vi "GeoData.vi"() -> ()   [LabVIEW 2017] (continued)
Ethridge\tTN\tGiles County\tH1\n38478\t47055\tPulaski\tTN\tGiles County\tH1\n38468\t47055\tLeoma\tTN\tGiles County\tH1\n38460\t47055\tGoodspring\tTN\tGiles County\tH1\n38477\t47055\tProspect\tTN\tGiles County\tH1\n37047\t47055\tCornersville\tTN\tGiles County\tH1\n38472\t47055\tLynnville\tTN\tGiles County\tH1\n38459\t47055\tFrankewing\tTN\tGiles County\tH1\n38451\t47055\tCulleoka\tTN\tGiles County\tH1\n38464\t47055\tLawrenceburg\tTN\tGiles County\tH1\n38483\t47055\tSummertown\tTN\tGiles County\tH1\n38473\t47055\tMinor hill\tTN\tGiles County\tH1\n38453\t47055\tDellrose\tTN\tGiles County\tH1\n38455\t47055\tElkton\tTN\tGiles County\tH1\n37848\t47057\tPowder springs\tTN\tGrainger County\tH1\n37708\t47057\tBean station\tTN\tGrainger County\tH1\n37888\t47057\tWashburn\tTN\tGrainger County\tH1\n37861\t47057\tRutledge\tTN\tGrainger County\tH1\n37779\t47057\tLuttrell\tTN\tGrainger County\tH1\n37811\t47057\tMooresburg\tTN\tGrainger County\tH1\n37869\t47057\tSneedville\tTN\tGrainger County\tH1\n37709\t47057\tBlaine\tTN\tGrainger County\tH1\n37806\t47057\tMascot\tTN\tGrainger County\tH1\n37881\t47057\tThorn hill\tTN\tGrainger County\tH1\n37711\t47059\tBulls gap\tTN\tGreene County\tH1\n37810\t47059\tMohawk\tTN\tGreene County\tH1\n37641\t47059\tChuckey\tTN\tGreene County\tH1\n37745\t47059\tGreeneville\tTN\tGreene County\tH1\n37681\t47059\tLimestone\tTN\tGreene County\tH1\n37743\t47059\tGreeneville\tTN\tGreene County\tH1\n37616\t47059\tAfton\tTN\tGreene County\tH1\n37656\t47059\tFall branch\tTN\tGreene County\tH1\n37809\t47059\tMidway\tTN\tGreene County\tH1\n37857\t47059\tRogersville\tTN\tGreene County\tH1\n37818\t47059\tMosheim\tTN\tGreene County\tH1\n37365\t47061\tPalmer\tTN\tGrundy County\tH1\n37357\t47061\tMorrison\tTN\tGrundy County\tH1\n37397\t47061\tWhitwell\tTN\tGrundy County\tH1\n37366\t47061\tPelham\tTN\tGrundy County\tH1\n37339\t47061\tGruetli laager\tTN\tGrundy County\tH1\n37387\t47061\tTracy city\tTN\tGrundy County\tH1\n37313\t47061\tCoalmont\tTN\tGrundy County\tH1\n37374\t47061\tSequatchie\tTN\tGrundy County\tH1\n37356\t47061\tMonteagle\tTN\tGrundy County\tH1\n37110\t47061\tMcminnville\tTN\tGrundy County\tH1\n37301\t47061\tAltamont\tTN\tGrundy County\tH1\n37305\t47061\tBeersheba springs\tTN\tGrundy County\tH1\n37711\t47063\tBulls gap\tTN\tHamblen County\tH1\n37813\t47063\tMorristown\tTN\tHamblen County\tH1\n37877\t47063\tTalbott\tTN\tHamblen County\tH1\n37815\t47063\tMorristown\tTN\tHamblen County\tH1\n37891\t47063\tWhitesburg\tTN\tHamblen County\tH1\n37816\t47063\tMorristown\tTN\tHamblen County\tH1\n37814\t47063\tMorristown\tTN\tHamblen County\tH1\n37778\t47063\tLowland\tTN\tHamblen County\tH1\n37860\t47063\tRussellville\tTN\tHamblen County\tH1\n37890\t47063\tWhite pine\tTN\tHamblen County\tH1\n37341\t47065\tHarrison\tTN\tHamilton County\tH1\n37353\t47065\tMc donald\tTN\tHamilton County\tH1\n37379\t47065\tSoddy daisy\tTN\tHamilton County\tH1\n37311\t47065\tCleveland\tTN\tHamilton County\tH1\n37350\t47065\tLookout mountain\tTN\tHamilton County\tH1\n37338\t47065\tGraysville\tTN\tHamilton County\tH1\n37409\t47065\tChattanooga\tTN\tHamilton County\tH1\n37302\t47065\tApison\tTN\tHamilton County\tH1\n37416\t47065\tChattanooga\tTN\tHamilton County\tH1\n37421\t47065\tChattanooga\tTN\tHamilton County\tH1\n37450\t47065\tChattanooga\tTN\tHamilton County\tH1\n37308\t47065\tBirchwood\tTN\tHamilton County\tH1\n37403\t47065\tChattanooga\tTN\tHamilton County\tH1\n37406\t47065\tChattanooga\tTN\tHamilton County\tH1\n37410\t47065\tChattanooga\tTN\tHamilton County\tH1\n37415\t47065\tChattanooga\tTN\tHamilton County\tH1\n37404\t47065\tChattanooga\tTN\tHamilton County\tH1\n37304\t47065\tBakewell\tTN\tHamilton County\tH1\n37373\t47065\tSale creek\tTN\tHamilton County\tH1\n37402\t47065\tChattanooga\tTN\tHamilton County\tH1\n37405\t47065\tChattanooga\tTN\tHamilton County\tH1\n37401\t47065\tChattanooga\tTN\tHamilton County\tH1\n37315\t47065\tCollegedale\tTN\tHamilton County\tH1\n37407\t47065\tChattanooga\tTN\tHamilton County\tH1\n37384\t47065\tSoddy daisy\tTN\tHamilton County\tH1\n37336\t47065\tGeorgetown\tTN\tHamilton County\tH1\n37363\t47065\tOoltewah\tTN\tHamilton County\tH1\n37411\t47065\tChattanooga\tTN\tHamilton County\tH1\n37412\t47065\tChattanooga\tTN\tHamilton County\tH1\n37422\t47065\tChattanooga\tTN\tHamilton County\tH1\n37351\t47065\tLupton city\tTN\tHamilton County\tH1\n37343\t47065\tHixson\tTN\tHamilton County\tH1\n37377\t47065\tSignal mountain\tTN\tHamilton County\tH1\n37408\t47065\tChattanooga\tTN\tHamilton County\tH1\n37419\t47065\tChattanooga\tTN\tHamilton County\tH1\n37414\t47065\tChattanooga\tTN\tHamilton County\tH1\n37424\t47065\tChattanooga\tTN\tHamilton County\tH1\n37765\t47067\tKyles ford\tTN\tHancock County\tH1\n37731\t47067\tEidson\tTN\tHancock County\tH1\n37879\t47067\tTazewell\tTN\tHancock County\tH1\n37752\t47067\tHarrogate\tTN\tHancock County\tH1\n37869\t47067\tSneedville\tTN\tHancock County\tH1\n37881\t47067\tThorn hill\tTN\tHancock County\tH1\n38075\t47069\tWhiteville\tTN\tHardeman County\tH1\n38061\t47069\tPocahontas\tTN\tHardeman County\tH1\n38392\t47069\tMercer\tTN\tHardeman County\tH1\n38356\t47069\tMedon\tTN\tHardeman County\tH1\n38067\t47069\tSaulsbury\tTN\tHardeman County\tH1\n38039\t47069\tGrand junction\tTN\tHardeman County\tH1\n38042\t47069\tHickory valley\tTN\tHardeman County\tH1\n38340\t47069\tHenderson\tTN\tHardeman County\tH1\n38052\t47069\tMiddleton\tTN\tHardeman County\tH1\n38381\t47069\tToone\tTN\tHardeman County\tH1\n38008\t47069\tBolivar\tTN\tHardeman County\tH1\n38044\t47069\tHornsby\tTN\tHardeman County\tH1\n38371\t47071\tSardis\tTN\tHardin County\tH1\n38379\t47071\tStantonville\tTN\tHardin County\tH1\n38327\t47071\tCrump\tTN\tHardin County\tH1\n38370\t47071\tSaltillo\tTN\tHardin County\tH1\n38425\t47071\tClifton\tTN\tHardin County\tH1\n38372\t47071\tSavannah\tTN\tHardin County\tH1\n38475\t47071\tOlivehill\tTN\tHardin County\tH1\n38326\t47071\tCounce\tTN\tHardin County\tH1\n38376\t47071\tShiloh\tTN\tHardin County\tH1\n38310\t47071\tAdamsville\tTN\tHardin County\tH1\n38357\t47071\tMichie\tTN\tHardin County\tH1\n38361\t47071\tMorris chapel\tTN\tHardin County\tH1\n38359\t47071\tMilledgeville\tTN\tHardin County\tH1\n38365\t47071\tPickwick dam\tTN\tHardin County\tH1\n37711\t47073\tBulls gap\tTN\tHawkins County\tH1\n37891\t47073\tWhitesburg\tTN\tHawkins County\tH1\n37645\t47073\tMount carmel\tTN\tHawkins County\tH1\n37745\t47073\tGreeneville\tTN\tHawkins County\tH1\n37731\t47073\tEidson\tTN\tHawkins County\tH1\n37642\t47073\tChurch hill\tTN\tHawkins County\tH1\n37873\t47073\tSurgoinsville\tTN\tHawkins County\tH1\n37811\t47073\tMooresburg\tTN\tHawkins County\tH1\n37857\t47073\tRogersville\tTN\tHawkins County\tH1\n37869\t47073\tSneedville\tTN\tHawkins County\tH1\n37660\t47073\tKingsport\tTN\tHawkins County\tH1\n37881\t47073\tThorn hill\tTN\tHawkins County\tH1\n38063\t47075\tRipley\tTN\tHaywood County\tH1\n38068\t47075\tSomerville\tTN\tHaywood County\tH1\n38075\t47075\tWhiteville\tTN\tHaywood County\tH1\n38006\t47075\tBells\tTN\tHaywood County\tH1\n38392\t47075\tMercer\tTN\tHaywood County\tH1\n38037\t47075\tGates\tTN\tHaywood County\tH1\n38069\t47075\tStanton\tTN\tHaywood County\tH1\n38301\t47075\tJackson\tTN\tHaywood County\tH1\n38012\t47075\tBrownsville\tTN\tHaywood County\tH1\n38049\t47075\tMason\tTN\tHaywood County\tH1\n38371\t47077\tSardis\tTN\tHenderson County\tH1\n38352\t47077\tLuray\tTN\tHenderson County\tH1\n38328\t47077\tDarden\tTN\tHenderson County\tH1\n38390\t47077\tYuma\tTN\tHenderson County\tH1\n38341\t47077\tHolladay\tTN\tHenderson County\tH1\n38370\t47077\tSaltillo\tTN\tHenderson County\tH1\n38329\t47077\tDecaturville\tTN\tHenderson County\tH1\n38321\t47077\tCedar grove\tTN\tHenderson County\tH1\n38345\t47077\tHuron\tTN\tHenderson County\tH1\n38313\t47077\tBeech bluff\tTN\tHenderson County\tH1\n38388\t47077\tWildersville\tTN\tHenderson County\tH1\n38347\t47077\tJacks creek\tTN\tHenderson County\tH1\n38351\t47077\tLexington\tTN\tHenderson County\tH1\n38374\t47077\tScotts hill\tTN\tHenderson County\tH1\n38363\t47077\tParsons\tTN\tHenderson County\tH1\n38368\t47077\tReagan\tTN\tHenderson County\tH1\n38201\t47079\tMc kenzie\tTN\tHenry County\tH1\n38242\t47079\tParis\tTN\tHenry County\tH1\n38251\t47079\tPuryear\tTN\tHenry County\tH1\n38229\t47079\tGleason\tTN\tHenry County\tH1\n38236\t47079\tMansfield\tTN\tHenry County\tH1\n38222\t47079\tBuchanan\tTN\tHenry County\tH1\n38224\t47079\tCottage grove\tTN\tHenry County\tH1\n38223\t47079\tComo\tTN\tHenry County\tH1\n38231\t47079\tHenry\tTN\tHenry County\tH1\n38256\t47079\tSpringville\tTN\tHenry County\tH1\n38454\t47081\tDuck river\tTN\tHickman County\tH1\n37033\t47081\tCenterville\tTN\tHickman County\tH1\n37098\t47081\tLyles\tTN\tHickman County\tH1\n37137\t47081\tNunnelly\tTN\tHickman County\tH1\n37140\t47081\tOnly\tTN\tHickman County\tH1\n38462\t47081\tHohenwald\tTN\tHickman County\tH1\n37096\t47081\tLinden\tTN\tHickman County\tH1\n37097\t47081\tLobelville\tTN\tHickman County\tH1\n38487\t47081\tWilliamsport\tTN\tHickman County\tH1\n38476\t47081\tPrimm springs\tTN\tHickman County\tH1\n37025\t47081\tBon aqua\tTN\tHickman County\tH1\n37055\t47081\tDickson\tTN\tHickman County\tH1\n37101\t47081\tMc ewen\tTN\tHickman County\tH1\n38461\t47081\tHampshire\tTN\tHickman County\tH1\n37175\t47083\tStewart\tTN\tHouston County\tH1\n37061\t47083\tErin\tTN\tHouston County\tH1\n37178\t47083\tTennessee ridge\tTN\tHouston County\tH1\n37181\t47083\tVanleer\tTN\tHouston County\tH1\n37051\t47083\tCumberland furnace\tTN\tHouston County\tH1\n37185\t47083\tWaverly\tTN\tHouston County\tH1\n37050\t47083\tCumberland city\tTN\tHouston County\tH1\n37101\t47083\tMc ewen\tTN\tHouston County\tH1\n37061\t47085\tErin\tTN\tHumphreys County\tH1\n37078\t47085\tHurricane mills\tTN\tHumphreys County\tH1\n37097\t47085\tLobelville\tTN\tHumphreys County\tH1\n37134\t47085\tNew johnsonville\tTN\tHumphreys County\tH1\n37185\t47085\tWaverly\tTN\tHumphreys County\tH1\n37101\t47085\tMc ewen\tTN\tHumphreys County\tH1\n38551\t47087\tCelina\tTN\tJackson County\tH1\n38506\t47087\tCookeville\tTN\tJackson County\tH1\n38545\t47087\tBloomington springs\tTN\tJackson County\tH1\n38588\t47087\tWhitleyville\tTN\tJackson County\tH1\n38501\t47087\tCookeville\tTN\tJackson County\tH1\n37145\t47087\tPleasant shade\tTN\tJackson County\tH1\n38564\t47087\tGranville\tTN\tJackson County\tH1\n38568\t47087\tHilham\tTN\tJackson County\tH1\n37030\t47087\tCarthage\tTN\tJackson County\tH1\n37150\t47087\tRed boiling springs\tTN\tJackson County\tH1\n38562\t47087\tGainesboro\tTN\tJackson County\tH1\n37813\t47089\tMorristown\tTN\tJefferson County\tH1\n37877\t47089\tTalbott\tTN\tJefferson County\tH1\n37876\t47089\tSevierville\tTN\tJefferson County\tH1\n37821\t47089\tNewport\tTN\tJefferson County\tH1\n37764\t47089\tKodak\tTN\tJefferson County\tH1\n37725\t47089\tDandridge\tTN\tJefferson County\tH1\n37890\t47089\tWhite pine\tTN\tJefferson County\tH1\n37871\t47089\tStrawberry plains\tTN\tJefferson County\tH1\n37760\t47089\tJefferson city\tTN\tJefferson County\tH1\n37820\t47089\tNew market\tTN\tJefferson County\tH1\n37683\t47091\tMountain city\tTN\tJohnson County\tH1\n37680\t47091\tLaurel bloomery\tTN\tJohnson County\tH1\n37640\t47091\tButler\tTN\tJohnson County\tH1\n37688\t47091\tShady valley\tTN\tJohnson County\tH1\n37691\t47091\tTrade\tTN\tJohnson County\tH1\n37909\t47093\tKnoxville\tTN\tKnox County\tH1\n37938\t47093\tKnoxville\tTN\tKnox County\tH1\n37929\t47093\tKnoxville\tTN\tKnox County\tH1\n37914\t47093\tKnoxville\tTN\tKnox County\tH1\n37915\t47093\tKnoxville\tTN\tKnox County\tH1\n37950\t47093\tKnoxville\tTN\tKnox County\tH1\n37995\t47093\tKnoxville\tTN\tKnox County\tH1\n37771\t47093\tLenoir city\tTN\tKnox County\tH1\n37754\t47093\tHeiskell\tTN\tKnox County\tH1\n37902\t47093\tKnoxville\tTN\tKnox County\tH1\n37930\t47093\tKnoxville\tTN\tKnox County\tH1\n37997\t47093\tKnoxville\tTN\tKnox County\tH1\n37764\t47093\tKodak\tTN\tKnox County\tH1\n37912\t47093\tKnoxville\tTN\tKnox County\tH1\n37919\t47093\tKnoxville\tTN\tKnox County\tH1\n37901\t47093\tKnoxville\tTN\tKnox County\tH1\n37772\t47093\tLenoir city\tTN\tKnox County\tH1\n37920\t47093\tKnoxville\tTN\tKnox County\tH1\n37849\t47093\tPowell\tTN\tKnox County\tH1\n37922\t47093\tKnoxville\tTN\tKnox County\tH1\n37923\t47093\tKnoxville\tTN\tKnox County\tH1\n37924\t47093\tKnoxville\tTN\tKnox County\tH1\n37853\t47093\tRockford\tTN\tKnox County\tH1\n37939\t47093\tKnoxville\tTN\tKnox County\tH1\n37807\t47093\tMaynardville\tTN\tKnox County\tH1\n37931\t47093\tKnoxville\tTN\tKnox County\tH1\n37916\t47093\tKnoxville\tTN\tKnox County\tH1\n37927\t47093\tKnoxville\tTN\tKnox County\tH1\n37934\t47093\tKnoxville\tTN\tKnox County\tH1\n37779\t47093\tLuttrell\tTN\tKnox County\tH1\n37917\t47093\tKnoxville\tTN\tKnox County\tH1\n37871\t47093\tStrawberry plains\tTN\tKnox County\tH1\n37932\t47093\tKnoxville\tTN\tKnox County\tH1\n37933\t47093\tKnoxville\tTN\tKnox County\tH1\n37940\t47093\tKnoxville\tTN\tKnox County\tH1\n37996\t47093\tKnoxville\tTN\tKnox County\tH1\n37709\t47093\tBlaine\tTN\tKnox County\tH1\n37721\t47093\tCorryton\tTN\tKnox County\tH1\n37830\t47093\tOak ridge\tTN\tKnox County\tH1\n37806\t47093\tMascot\tTN\tKnox County\tH1\n37918\t47093\tKnoxville\tTN\tKnox County\tH1\n37921\t47093\tKnoxville\tTN\tKnox County\tH1\n37928\t47093\tKnoxville\tTN\tKnox County\tH1\n37998\t47093\tKnoxville\tTN\tKnox County\tH1\n38080\t47095\tRidgely\tTN\tLake County\tH1\n38077\t47095\tWynnburg\tTN\tLake County\tH1\n38079\t47095\tTiptonville\tTN\tLake County\tH1\n38063\t47097\tRipley\tTN\tLauderdale County\tH1\n38037\t47097\tGates\tTN\tLauderdale County\tH1\n38040\t47097\tHalls\tTN\tLauderdale County\tH1\n38041\t47097\tHenning\tTN\tLauderdale County\tH1\n38469\t47099\tLoretto\tTN\tLawrence County\tH1\n38474\t47099\tMount pleasant\tTN\tLawrence County\tH1\n38463\t47099\tIron city\tTN\tLawrence County\tH1\n38486\t47099\tWestpoint\tTN\tLawrence County\tH1\n38456\t47099\tEthridge\tTN\tLawrence County\tH1\n38481\t47099\tSaint joseph\tTN\tLawrence County\tH1\n38468\t47099\tLeoma\tTN\tLawrence County\tH1\n38457\t47099\tFive points\tTN\tLawrence County\tH1\n38464\t47099\tLawrenceburg\tTN\tLawrence County\tH1\n38483\t47099\tSummertown\tTN\tLawrence County\tH1\n38473\t47099\tMinor hill\tTN\tLawrence County\tH1\n38474\t47101\tMount pleasant\tTN\tLewis County\tH1\n38462\t47101\tHohenwald\tTN\tLewis County\tH1\n37096\t47101\tLinden\tTN\tLewis County\tH1\n38485\t47101\tWaynesboro\tTN\tLewis County\tH1\n38483\t47101\tSummertown\tTN\tLewis County\tH1\n38461\t47101\tHampshire\tTN\tLewis County\tH1\n38488\t47103\tTaft\tTN\tLincoln County\tH1\n37328\t47103\tElora\tTN\tLincoln County\tH1\n37334\t47103\tFayetteville\tTN\tLincoln County\tH1\n38449\t47103\tArdmore\tTN\tLincoln County\tH1\n37144\t47103\tPetersburg\tTN\tLincoln County\tH1\n38478\t47103\tPulaski\tTN\tLincoln County\tH1\n37345\t47103\tHuntland\tTN\tLincoln County\tH1\n37335\t47103\tFlintville\tTN\tLincoln County\tH1\n37047\t47103\tCornersville\tTN\tLincoln County\tH1\n38459\t47103\tFrankewing\tTN\tLincoln County\tH1\n37348\t47103\tKelso\tTN\tLincoln County\tH1\n37359\t47103\tMulberry\tTN\tLincoln County\tH1\n38453\t47103\tDellrose\tTN\tLincoln County\tH1\n37885\t47105\tVonore\tTN\tLoudon County\tH1\n37737\t47105\tFriendsville\tTN\tLoudon County\tH1\n37771\t47105\tLenoir city\tTN\tLoudon County\tH1\n37846\t47105\tPhiladelphia\tTN\tLoudon County\tH1\n37772\t47105\tLenoir city\tTN\tLoudon County\tH1\n37801\t47105\tMaryville\tTN\tLoudon County\tH1\n37922\t47105\tKnoxville\tTN\tLoudon County\tH1\n37874\t47105\tSweetwater\tTN\tLoudon County\tH1\n37774\t47105\tLoudon\tTN\tLoudon County\tH1\n37742\t47105\tGreenback\tTN\tLoudon County\tH1\n37880\t47107\tTen mile\tTN\tMcMinn County\tH1\n37331\t47107\tEtowah\tTN\tMcMinn County\tH1\n37329\t47107\tEnglewood\tTN\tMcMinn County\tH1\n37846\t47107\tPhiladelphia\tTN\tMcMinn County\tH1\n37354\t47107\tMadisonville\tTN\tMcMinn County\tH1\n37322\t47107\tDecatur\tTN\tMcMinn County\tH1\n37371\t47107\tAthens\tTN\tMcMinn County\tH1\n37325\t47107\tDelano\tTN\tMcMinn County\tH1\n37370\t47107\tRiceville\tTN\tMcMinn County\tH1\n37874\t47107\tSweetwater\tTN\tMcMinn County\tH1\n37303\t47107\tAthens\tTN\tMcMinn County\tH1\n37309\t47107\tCalhoun\tTN\tMcMinn County\tH1\n37826\t47107\tNiota\tTN\tMcMinn County\tH1\n38379\t47109\tStantonville\tTN\tMcNairy County\tH1\n38061\t47109\tPocahontas\tTN\tMcNairy County\tH1\n38339\t47109\tGuys\tTN\tMcNairy County\tH1\n38393\t47109\tChewalla\tTN\tMcNairy County\tH1\n38375\t47109\tSelmer\tTN\tMcNairy County\tH1\n38332\t47109\tEnville\tTN\tMcNairy County\tH1\n38376\t47109\tShiloh\tTN\tMcNairy County\tH1\n38310\t47109\tAdamsville\tTN\tMcNairy County\tH1\n38334\t47109\tFinger\tTN\tMcNairy County\tH1\n38357\t47109\tMichie\tTN\tMcNairy County\tH1\n38367\t47109\tRamer\tTN\tMcNairy County\tH1\n38361\t47109\tMorris chapel\tTN\tMcNairy County\tH1\n38315\t47109\tBethel springs\tTN\tMcNairy County\tH1\n38359\t47109\tMilledgeville\tTN\tMcNairy County\tH1\n38044\t47109\tHornsby\tTN\tMcNairy County\tH1\n37074\t47111\tHartsville\tTN\tMacon County\tH1\n37022\t47111\tBethpage\tTN\tMacon County\tH1\n37083\t47111\tLafayette\tTN\tMacon County\tH1\n37186\t47111\tWestmoreland\tTN\tMacon County\tH1\n37057\t47111\tDixon springs\tTN\tMacon County\tH1\n38588\t47111\tWhitleyville\tTN\tMacon County\tH1\n38575\t47111\tMoss\tTN\tMacon County\tH1\n37145\t47111\tPleasant shade\tTN\tMacon County\tH1\n37150\t47111\tRed boiling springs\tTN\tMacon County\tH1\n38006\t47113\tBells\tTN\tMadison County\tH1\n38303\t47113\tJackson\tTN\tMadison County\tH1\n38378\t47113\tSpring creek\tTN\tMadison County\tH1\n38392\t47113\tMercer\tTN\tMadison County\tH1\n38366\t47113\tPinson\tTN\tMadison County\tH1\n38305\t47113\tJackson\tTN\tMadison County\tH1\n38301\t47113\tJackson\tTN\tMadison County\tH1\n38356\t47113\tMedon\tTN\tMadison County\tH1\n38302\t47113\tJackson\tTN\tMadison County\tH1\n38348\t47113\tLavinia\tTN\tMadison County\tH1\n38313\t47113\tBeech bluff\tTN\tMadison County\tH1\n38362\t47113\tOakfield\tTN\tMadison County\tH1\n38351\t47113\tLexington\tTN\tMadison County\tH1\n38343\t47113\tHumboldt\tTN\tMadison County\tH1\n38308\t47113\tJackson\tTN\tMadison County\tH1\n38355\t47113\tMedina\tTN\tMadison County\tH1\n38391\t47113\tDenmark\tTN\tMadison County\tH1\n37365\t47115\tPalmer\tTN\tMarion County\tH1\n37340\t47115\tGuild\tTN\tMarion County\tH1\n37397\t47115\tWhitwell\tTN\tMarion County\tH1\n37366\t47115\tPelham\tTN\tMarion County\tH1\n37347\t47115\tJasper\tTN\tMarion County\tH1\n37387\t47115\tTracy city\tTN\tMarion County\tH1\n37405\t47115\tChattanooga\tTN\tMarion County\tH1\n37396\t47115\tWhiteside\tTN\tMarion County\tH1\n37374\t47115\tSequatchie\tTN\tMarion County\tH1\n37380\t47115\tSouth pittsburg\tTN\tMarion County\tH1\n37375\t47115\tSewanee\tTN\tMarion County\tH1\n37356\t47115\tMonteagle\tTN\tMarion County\tH1\n37377\t47115\tSignal mountain\tTN\tMarion County\tH1\n37419\t47115\tChattanooga\tTN\tMarion County\tH1\n37060\t47117\tEagleville\tTN\tMarshall County\tH1\n37034\t47117\tChapel hill\tTN\tMarshall County\tH1\n37144\t47117\tPetersburg\tTN\tMarshall County\tH1\n37174\t47117\tSpring hill\tTN\tMarshall County\tH1\n37091\t47117\tLewisburg\tTN\tMarshall County\tH1\n37019\t47117\tBelfast\tTN\tMarshall County\tH1\n37046\t47117\tCollege grove\tTN\tMarshall County\tH1\n38401\t47117\tColumbia\tTN\tMarshall County\tH1\n37180\t47117\tUnionville\tTN\tMarshall County\tH1\n37047\t47117\tCornersville\tTN\tMarshall County\tH1\n38472\t47117\tLynnville\tTN\tMarshall County\tH1\n38451\t47117\tCulleoka\tTN\tMarshall County\tH1\n38474\t47119\tMount pleasant\tTN\tMaury County\tH1\n38454\t47119\tDuck river\tTN\tMaury County\tH1\n37174\t47119\tSpring hill\tTN\tMaury County\tH1\n37091\t47119\tLewisburg\tTN\tMaury County\tH1\n38482\t47119\tSanta fe\tTN\tMaury County\tH1\n38487\t47119\tWilliamsport\tTN\tMaury County\tH1\n38401\t47119\tColumbia\tTN\tMaury County\tH1\n38472\t47119\tLynnville\tTN\tMaury County\tH1\n38476\t47119\tPrimm springs\tTN\tMaury County\tH1\n38451\t47119\tCulleoka\tTN\tMaury County\tH1\n38483\t47119\tSummertown\tTN\tMaury County\tH1\n38402\t47119\tColumbia\tTN\tMaury County\tH1\n38461\t47119\tHampshire\tTN\tMaury County\tH1\n37880\t47121\tTen mile\tTN\tMeigs County\tH1\n37308\t47121\tBirchwood\tTN\tMeigs County\tH1\n37846\t47121\tPhiladelphia\tTN\tMeigs County\tH1\n37322\t47121\tDecatur\tTN\tMeigs County\tH1\n37336\t47121\tGeorgetown\tTN\tMeigs County\tH1\n37321\t47121\tDayton\tTN\tMeigs County\tH1\n37826\t47121\tNiota\tTN\tMeigs County\tH1\n37385\t47123\tTellico plains\tTN\tMonroe County\tH1\n37885\t47123\tVonore\tTN\tMonroe County\tH1\n37369\t47123\tReliance\tTN\tMonroe County\tH1\n37329\t47123\tEnglewood\tTN\tMonroe County\tH1\n37846\t47123\tPhiladelphia\tTN\tMonroe County\tH1\n37354\t47123\tMadisonville\tTN\tMonroe County\tH1\n37801\t47123\tMaryville\tTN\tMonroe County\tH1\n37874\t47123\tSweetwater\tTN\tMonroe County\tH1\n37314\t47123\tCoker creek\tTN\tMonroe County\tH1\n37774\t47123\tLoudon\tTN\tMonroe County\tH1\n37052\t47125\tCunningham\tTN\tMontgomery County\tH1\n37041\t47125\tClarksville\tTN\tMontgomery County\tH1\n37061\t47125\tErin\tTN\tMontgomery County\tH1\n37079\t47125\tIndian mound\tTN\tMontgomery County\tH1\n37044\t47125\tClarksville\tTN\tMontgomery County\tH1\n37015\t47125\tAshland city\tTN\tMontgomery County\tH1\n37043\t47125\tClarksville\tTN\tMontgomery County\tH1\n37035\t47125\tChapmansboro\tTN\tMontgomery County\tH1\n37032\t47125\tCedar hill\tTN\tMontgomery County\tH1\n37142\t47125\tPalmyra\tTN\tMontgomery County\tH1\n37042\t47125\tClarksville\tTN\tMontgomery County\tH1\n37171\t47125\tSouthside\tTN\tMontgomery County\tH1\n37010\t47125\tAdams\tTN\tMontgomery County\tH1\n37040\t47125\tClarksville\tTN\tMontgomery County\tH1\n37051\t47125\tCumberland furnace\tTN\tMontgomery County\tH1\n37191\t47125\tWoodlawn\tTN\tMontgomery County\tH1\n37050\t47125\tCumberland city\tTN\tMontgomery County\tH1\n42223\t47125\tFort campbell\tTN\tMontgomery County\tH1\n37352\t47127\tLynchburg\tTN\tMoore County\tH6\n37334\t47127\tFayetteville\tTN\tMoore County\tH6\n37183\t47127\tWartrace\tTN\tMoore County\tH6\n37144\t47127\tPetersburg\tTN\tMoore County\tH6\n37388\t47127\tTullahoma\tTN\tMoore County\tH6\n37398\t47127\tWinchester\tTN\tMoore County\tH6\n37306\t47127\tBelvidere\tTN\tMoore County\tH6\n37160\t47127\tShelbyville\tTN\tMoore County\tH6\n37360\t47127\tNormandy\tTN\tMoore County\tH6\n37359\t47127\tMulberry\tTN\tMoore County\tH6\n37872\t47129\tSunbright\tTN\tMorgan County\tH1\n37829\t47129\tOakdale\tTN\tMorgan County\tH1\n37733\t47129\tRugby\tTN\tMorgan County\tH1\n37840\t47129\tOliver springs\tTN\tMorgan County\tH1\n37854\t47129\tRockwood\tTN\tMorgan County\tH1\n37887\t47129\tWartburg\tTN\tMorgan County\tH1\n37845\t47129\tPetros\tTN\tMorgan County\tH1\n37726\t47129\tDeer lodge\tTN\tMorgan County\tH1\n37852\t47129\tRobbins\tTN\tMorgan County\tH1\n37719\t47129\tCoalfield\tTN\tMorgan County\tH1\n37748\t47129\tHarriman\tTN\tMorgan County\tH1\n37770\t47129\tLancing\tTN\tMorgan County\tH1\n38271\t47131\tWoodland mills\tTN\tObion County\tH1\n38255\t47131\tSharon\tTN\tObion County\tH1\n38240\t47131\tObion\tTN\tObion County\tH1\n38237\t47131\tMartin\tTN\tObion County\tH1\n38233\t47131\tKenton\tTN\tObion County\tH1\n38260\t47131\tTroy\tTN\tObion County\tH1\n38253\t47131\tRives\tTN\tObion County\tH1\n38080\t47131\tRidgely\tTN\tObion County\tH1\n38254\t47131\tSamburg\tTN\tObion County\tH1\n38261\t47131\tUnion city\tTN\tObion County\tH1\n38257\t47131\tSouth fulton\tTN\tObion County\tH1\n38232\t47131\tHornbeak\tTN\tObion County\tH1\n38079\t47131\tTiptonville\tTN\tObion County\tH1\n38259\t47131\tTrimble\tTN\tObion County\tH1\n38281\t47131\tUnion city\tTN\tObion County\tH1\n38580\t47133\tRickman\tTN\tOverton County\tH1\n38551\t47133\tCelina\tTN\tOverton County\tH1\n38506\t47133\tCookeville\tTN\tOverton County\tH1\n38543\t47133\tAlpine\tTN\tOverton County\tH1\n38589\t47133\tWilder\tTN\tOverton County\tH1\n38570\t47133\tLivingston\tTN\tOverton County\tH1\n38553\t47133\tClarkrange\tTN\tOverton County\tH1\n38541\t47133\tAllons\tTN\tOverton County\tH1\n38542\t47133\tAllred\tTN\tOverton County\tH1\n38501\t47133\tCookeville\tTN\tOverton County\tH1\n38574\t47133\tMonterey\tTN\tOverton County\tH1\n38568\t47133\tHilham\tTN\tOverton County\tH1\n38573\t47133\tMonroe\tTN\tOverton County\tH1\n38554\t47133\tCrawford\tTN\tOverton County\tH1\n37033\t47135\tCenterville\tTN\tPerry County\tH1\n38425\t47135\tClifton\tTN\tPerry County\tH1\n37096\t47135\tLinden\tTN\tPerry County\tH1\n37097\t47135\tLobelville\tTN\tPerry County\tH1\n38543\t47137\tAlpine\tTN\tPickett County\tH1\n38556\t47137\tJamestown\tTN\tPickett County\tH1\n38549\t47137\tByrdstown\tTN\tPickett County\tH1\n38577\t47137\tPall mall\tTN\tPickett County\tH1\n38573\t47137\tMonroe\tTN\tPickett County\tH1\n37307\t47139\tBenton\tTN\tPolk County\tH1\n37385\t47139\tTellico plains\tTN\tPolk County\tH1\n37362\t47139\tOld fort\tTN\tPolk County\tH1\n37361\t47139\tOcoee\tTN\tPolk County\tH1\n37369\t47139\tReliance\tTN\tPolk County\tH1\n37310\t47139\tCharleston\tTN\tPolk County\tH1\n37317\t47139\tCopperhill\tTN\tPolk County\tH1\n37333\t47139\tFarner\tTN\tPolk County\tH1\n37323\t47139\tCleveland\tTN\tPolk County\tH1\n37325\t47139\tDelano\tTN\tPolk County\tH1\n37391\t47139\tTurtletown\tTN\tPolk County\tH1\n37309\t47139\tCalhoun\tTN\tPolk County\tH1\n37326\t47139\tDucktown\tTN\tPolk County\tH1\n38506\t47141\tCookeville\tTN\tPutnam County\tH1\n38545\t47141\tBloomington springs\tTN\tPutnam County\tH1\n38583\t47141\tSparta\tTN\tPutnam County\tH1\n38552\t47141\tChestnut mound\tTN\tPutnam County\tH1\n38582\t47141\tSilver point\tTN\tPutnam County\tH1\n38503\t47141\tCookeville\tTN\tPutnam County\tH1\n38501\t47141\tCookeville\tTN\tPutnam County\tH1\n38502\t47141\tCookeville\tTN\tPutnam County\tH1\n38564\t47141\tGranville\tTN\tPutnam County\tH1\n38574\t47141\tMonterey\tTN\tPutnam County\tH1\n38548\t47141\tBuffalo valley\tTN\tPutnam County\tH1\n38544\t47141\tBaxter\tTN\tPutnam County\tH1\n37381\t47143\tSpring city\tTN\tRhea County\tH1\n37338\t47143\tGraysville\tTN\tRhea County\tH1\n37367\t47143\tPikeville\tTN\tRhea County\tH1\n37332\t47143\tEvensville\tTN\tRhea County\tH1\n37337\t47143\tGrandview\tTN\tRhea County\tH1\n37373\t47143\tSale creek\tTN\tRhea County\tH1\n37321\t47143\tDayton\tTN\tRhea County\tH1\n37880\t47145\tTen mile\tTN\tRoane County\tH1\n37771\t47145\tLenoir city\tTN\tRoane County\tH1\n37846\t47145\tPhiladelphia\tTN\tRoane County\tH1\n37763\t47145\tKingston\tTN\tRoane County\tH1\n37840\t47145\tOliver springs\tTN\tRoane County\tH1\n37874\t47145\tSweetwater\tTN\tRoane County\tH1\n37854\t47145\tRockwood\tTN\tRoane County\tH1\n37748\t47145\tHarriman\tTN\tRoane County\tH1\n37774\t47145\tLoudon\tTN\tRoane County\tH1\n37830\t47145\tOak ridge\tTN\tRoane County\tH1\n37073\t47147\tGreenbrier\tTN\tRobertson County\tH1\n37141\t47147\tOrlinda\tTN\tRobertson County\tH1\n37048\t47147\tCottontown\tTN\tRobertson County\tH1\n37172\t47147\tSpringfield\tTN\tRobertson County\tH1\n37072\t47147\tGoodlettsville\tTN\tRobertson County\tH1\n37043\t47147\tClarksville\tTN\tRobertson County\tH1\n37188\t47147\tWhite house\tTN\tRobertson County\tH1\n37032\t47147\tCedar hill\tTN\tRobertson County\tH1\n37148\t47147\tPortland\tTN\tRobertson County\tH1\n37152\t47147\tRidgetop\tTN\tRobertson County\tH1\n37146\t47147\tPleasant view\tTN\tRobertson County\tH1\n37010\t47147\tAdams\tTN\tRobertson County\tH1\n37049\t47147\tCross plains\tTN\tRobertson County\tH1\n37080\t47147\tJoelton\tTN\tRobertson County\tH1\n37060\t47149\tEagleville\tTN\tRutherford County\tH1\n37153\t47149\tRockvale\tTN\tRutherford County\tH1\n37086\t47149\tLa vergne\tTN\tRutherford County\tH1\n37129\t47149\tMurfreesboro\tTN\tRutherford County\tH1\n37118\t47149\tMilton\tTN\tRutherford County\tH1\n37063\t47149\tFosterville\tTN\tRutherford County\tH1\n37131\t47149\tMurfreesboro\tTN\tRutherford County\tH1\n37020\t47149\tBell buckle\tTN\tRutherford County\tH1\n37090\t47149\tLebanon\tTN\tRutherford County\tH1\n37037\t47149\tChristiana\tTN\tRutherford County\tH1\n37014\t47149\tArrington\tTN\tRutherford County\tH1\n37122\t47149\tMount juliet\tTN\tRutherford County\tH1\n37135\t47149\tNolensville\tTN\tRutherford County\tH1\n37128\t47149\tMurfreesboro\tTN\tRutherford County\tH1\n37089\t47149\tLa vergne\tTN\tRutherford County\tH1\n37149\t47149\tReadyville\tTN\tRutherford County\tH1\n37046\t47149\tCollege grove\tTN\tRutherford County\tH1\n37180\t47149\tUnionville\tTN\tRutherford County\tH1\n37133\t47149\tMurfreesboro\tTN\tRutherford County\tH1\n37160\t47149\tShelbyville\tTN\tRutherford County\tH1\n37130\t47149\tMurfreesboro\tTN\tRutherford County\tH1\n37167\t47149\tSmyrna\tTN\tRutherford County\tH1\n37127\t47149\tMurfreesboro\tTN\tRutherford County\tH1\n37085\t47149\tLascassas\tTN\tRutherford County\tH1\n37132\t47149\tMurfreesboro\tTN\tRutherford County\tH1\n37755\t47151\tHelenwood\tTN\tScott County\tH1\n37841\t47151\tOneida\tTN\tScott County\tH1\n37872\t47151\tSunbright\tTN\tScott County\tH1\n37756\t47151\tHuntsville\tTN\tScott County\tH1\n38504\t47151\tAllardt\tTN\tScott County\tH1\n37847\t47151\tPioneer\tTN\tScott County\tH1\n37732\t47151\tElgin\tTN\tScott County\tH1\n37852\t47151\tRobbins\tTN\tScott County\tH1\n37892\t47151\tWinfield\tTN\tScott County\tH1\n37379\t47153\tSoddy daisy\tTN\tSequatchie County\tH1\n37365\t47153\tPalmer\tTN\tSequatchie County\tH1\n37338\t47153\tGraysville\tTN\tSequatchie County\tH1\n37367\t47153\tPikeville\tTN\tSequatchie County\tH1\n37397\t47153\tWhitwell\tTN\tSequatchie County\tH1\n37327\t47153\tDunlap\tTN\tSequatchie County\tH1\n37110\t47153\tMcminnville\tTN\tSequatchie County\tH1\n37377\t47153\tSignal mountain\tTN\tSequatchie County\tH1\n37865\t47155\tSeymour\tTN\tSevier County\tH1\n37738\t47155\tGatlinburg\tTN\tSevier County\tH1\n37876\t47155\tSevierville\tTN\tSevier County\tH1\n37722\t47155\tCosby\tTN\tSevier County\tH1\n37864\t47155\tSevierville\tTN\tSevier County\tH1\n37764\t47155\tKodak\tTN\tSevier County\tH1\n37862\t47155\tSevierville\tTN\tSevier County\tH1\n37920\t47155\tKnoxville\tTN\tSevier County\tH1\n37725\t47155\tDandridge\tTN\tSevier County\tH1\n37868\t47155\tPigeon forge\tTN\tSevier County\tH1\n37863\t47155\tPigeon forge\tTN\tSevier County\tH1\n37871\t47155\tStrawberry plains\tTN\tSevier County\tH1\n37820\t47155\tNew market\tTN\tSevier County\tH1\n38134\t47157\tMemphis\tTN\tShelby County\tH1\n38182\t47157\tMemphis\tTN\tShelby County\tH1\n38112\t47157\tMemphis\tTN\tShelby County\tH1\n38117\t47157\tMemphis\tTN\tShelby County\tH1\n38137\t47157\tMemphis\tTN\tShelby County\tH1\n38017\t47157\tCollierville\tTN\tShelby County\tH1\n38111\t47157\tMemphis\tTN\tShelby County\tH1\n38167\t47157\tMemphis\tTN\tShelby County\tH1\n38193\t47157\tMemphis\tTN\tShelby County\tH1\n38120\t47157\tMemphis\tTN\tShelby County\tH1\n38133\t47157\tMemphis\tTN\tShelby County\tH1\n38138\t47157\tGermantown\tTN\tShelby County\tH1\n38107\t47157\tMemphis\tTN\tShelby County\tH1\n38109\t47157\tMemphis\tTN\tShelby County\tH1\n38104\t47157\tMemphis\tTN\tShelby County\tH1\n38152\t47157\tMemphis\tTN\tShelby County\tH1\n37501\t47157\tMemphis\tTN\tShelby County\tH1\n38125\t47157\tMemphis\tTN\tShelby County\tH1\n38004\t47157\tAtoka\tTN\tShelby County\tH1\n38018\t47157\tCordova\tTN\tShelby County\tH1\n38011\t47157\tBrighton\tTN\tShelby County\tH1\n38130\t47157\tMemphis\tTN\tShelby County\tH1\n38168\t47157\tMemphis\tTN\tShelby County\tH1\n38161\t47157\tMemphis\tTN\tShelby County\tH1\n38114\t47157\tMemphis\tTN\tShelby County\tH1\n38126\t47157\tMemphis\tTN\tShelby County\tH1\n38027\t47157\tCollierville\tTN\tShelby County\tH1\n38002\t47157\tArlington\tTN\tShelby County\tH1\n38173\t47157\tMemphis\tTN\tShelby County\tH1\n38014\t47157\tBrunswick\tTN\tShelby County\tH1\n38119\t47157\tMemphis\tTN\tShelby County\tH1\n38127\t47157\tMemphis\tTN\tShelby County\tH1\n38122\t47157\tMemphis\tTN\tShelby County\tH1\n38141\t47157\tMemphis\tTN\tShelby County\tH1\n38174\t47157\tMemphis\tTN\tShelby County\tH1\n38108\t47157\tMemphis\tTN\tShelby County\tH1\n38183\t47157\tGermantown\tTN\tShelby County\tH1\n38187\t47157\tMemphis\tTN\tShelby County\tH1\n38188\t47157\tMemphis\tTN\tShelby County\tH1\n38118\t47157\tMemphis\tTN\tShelby County\tH1\n38116\t47157\tMemphis\tTN\tShelby County\tH1\n38157\t47157\tMemphis\tTN\tShelby County\tH1\n38016\t47157\tCordova\tTN\tShelby County\tH1\n38177\t47157\tMemphis\tTN\tShelby County\tH1\n38181\t47157\tMemphis\tTN\tShelby County\tH1\n38166\t47157\tMemphis\tTN\tShelby County\tH1\n38139\t47157\tGermantown\tTN\tShelby County\tH1\n38175\t47157\tMemphis\tTN\tShelby County\tH1\n38053\t47157\tMillington\tTN\tShelby County\tH1\n38105\t47157\tMemphis\tTN\tShelby County\tH1\n38088\t47157\tCordova\tTN\tShelby County\tH1\n38083\t47157\tMillington\tTN\tShelby County\tH1\n38124\t47157\tMemphis\tTN\tShelby County\tH1\n38101\t47157\tMemphis\tTN\tShelby County\tH1\n38190\t47157\tMemphis\tTN\tShelby County\tH1\n38186\t47157\tMemphis\tTN\tShelby County\tH1\n38132\t47157\tMemphis\tTN\tShelby County\tH1\n38136\t47157\tMemphis\tTN\tShelby County\tH1\n38054\t47157\tMillington\tTN\tShelby County\tH1\n38197\t47157\tMemphis\tTN\tShelby County\tH1\n38055\t47157\tMillington\tTN\tShelby County\tH1\n38128\t47157\tMemphis\tTN\tShelby County\tH1\n38135\t47157\tMemphis\tTN\tShelby County\tH1\n38115\t47157\tMemphis\tTN\tShelby County\tH1\n38106\t47157\tMemphis\tTN\tShelby County\tH1\n38028\t47157\tEads\tTN\tShelby County\tH1\n38103\t47157\tMemphis\tTN\tShelby County\tH1\n38029\t47157\tEllendale\tTN\tShelby County\tH1\n38131\t47157\tMemphis\tTN\tShelby County\tH1\n38184\t47157\tMemphis\tTN\tShelby County\tH1\n38113\t47157\tMemphis\tTN\tShelby County\tH1\n37074\t47159\tHartsville\tTN\tSmith County\tH1\n38563\t47159\tGordonsville\tTN\tSmith County\tH1\n38567\t47159\tHickman\tTN\tSmith County\tH1\n38552\t47159\tChestnut mound\tTN\tSmith County\tH1\n37090\t47159\tLebanon\tTN\tSmith County\tH1\n38569\t47159\tLancaster\tTN\tSmith County\tH1\n38560\t47159\tElmwood\tTN\tSmith County\tH1\n37057\t47159\tDixon springs\tTN\tSmith County\tH1\n37145\t47159\tPleasant shade\tTN\tSmith County\tH1\n38547\t47159\tBrush creek\tTN\tSmith County\tH1\n37012\t47159\tAlexandria\tTN\tSmith County\tH1\n37151\t47159\tRiddleton\tTN\tSmith County\tH1\n37184\t47159\tWatertown\tTN\tSmith County\tH1\n37030\t47159\tCarthage\tTN\tSmith County\tH1\n37087\t47159\tLebanon\tTN\tSmith County\tH1\n38548\t47159\tBuffalo valley\tTN\tSmith County\tH1\n37175\t47161\tStewart\tTN\tStewart County\tH1\n37061\t47161\tErin\tTN\tStewart County\tH1\n37079\t47161\tIndian mound\tTN\tStewart County\tH1\n37178\t47161\tTennessee ridge\tTN\tStewart County\tH1\n37023\t47161\tBig rock\tTN\tStewart County\tH1\n37028\t47161\tBumpus mills\tTN\tStewart County\tH1\n37058\t47161\tDover\tTN\tStewart County\tH1\n37050\t47161\tCumberland city\tTN\tStewart County\tH1\n37659\t47163\tJonesborough\tTN\tSullivan County\tH1\n37669\t47163\tKingsport\tTN\tSullivan County\tH1\n37662\t47163\tKingsport\tTN\tSullivan County\tH1\n37615\t47163\tJohnson city\tTN\tSullivan County\tH1\n37617\t47163\tBlountville\tTN\tSullivan County\tH1\n37618\t47163\tBluff city\tTN\tSullivan County\tH1\n37694\t47163\tWatauga\tTN\tSullivan County\tH1\n37625\t47163\tBristol\tTN\tSullivan County\tH1\n37620\t47163\tBristol\tTN\tSullivan County\tH1\n37663\t47163\tKingsport\tTN\tSullivan County\tH1\n37656\t47163\tFall branch\tTN\tSullivan County\tH1\n37686\t47163\tPiney flats\tTN\tSullivan County\tH1\n37665\t47163\tKingsport\tTN\tSullivan County\tH1\n37857\t47163\tRogersville\tTN\tSullivan County\tH1\n37660\t47163\tKingsport\tTN\tSullivan County\tH1\n37664\t47163\tKingsport\tTN\tSullivan County\tH1\n37621\t47163\tBristol\tTN\tSullivan County\tH1\n37699\t47163\tPiney flats\tTN\tSullivan County\tH1\n37077\t47165\tHendersonville\tTN\tSumner County\tH1\n37022\t47165\tBethpage\tTN\tSumner County\tH1\n37073\t47165\tGreenbrier\tTN\tSumner County\tH1\n37048\t47165\tCottontown\tTN\tSumner County\tH1\n37186\t47165\tWestmoreland\tTN\tSumner County\tH1\n37072\t47165\tGoodlettsville\tTN\tSumner County\tH1\n37066\t47165\tGallatin\tTN\tSumner County\tH1\n37031\t47165\tCastalian springs\tTN\tSumner County\tH1\n37188\t47165\tWhite house\tTN\tSumner County\tH1\n37148\t47165\tPortland\tTN\tSumner County\tH1\n37049\t47165\tCross plains\tTN\tSumner County\tH1\n37075\t47165\tHendersonville\tTN\tSumner County\tH1\n37119\t47165\tMitchellville\tTN\tSumner County\tH1\n38069\t47167\tStanton\tTN\tTipton County\tH1\n38058\t47167\tMunford\tTN\tTipton County\tH1\n38004\t47167\tAtoka\tTN\tTipton County\tH1\n38011\t47167\tBrighton\tTN\tTipton County\tH1\n38023\t47167\tDrummonds\tTN\tTipton County\tH1\n38049\t47167\tMason\tTN\tTipton County\tH1\n38015\t47167\tBurlison\tTN\tTipton County\tH1\n38071\t47167\tTipton\tTN\tTipton County\tH1\n38019\t47167\tCovington\tTN\tTipton County\tH1\n38053\t47167\tMillington\tTN\tTipton County\tH1\n37074\t47169\tHartsville\tTN\tTrousdale County\tH6\n37022\t47169\tBethpage\tTN\tTrousdale County\tH6\n37031\t47169\tCastalian springs\tTN\tTrousdale County\tH6\n37057\t47169\tDixon springs\tTN\tTrousdale County\tH6\n37087\t47169\tLebanon\tTN\tTrousdale County\tH6\n37657\t47171\tFlag pond\tTN\tUnicoi County\tH1\n37658\t47171\tHampton\tTN\tUnicoi County\tH1\n37601\t47171\tJohnson city\tTN\tUnicoi County\tH1\n37692\t47171\tUnicoi\tTN\tUnicoi County\tH1\n37650\t47171\tErwin\tTN\tUnicoi County\tH1\n37643\t47171\tElizabethton\tTN\tUnicoi County\tH1\n37938\t47173\tKnoxville\tTN\tUnion County\tH1\n37848\t47173\tPowder springs\tTN\tUnion County\tH1\n37705\t47173\tAndersonville\tTN\tUnion County\tH1\n37754\t47173\tHeiskell\tTN\tUnion County\tH1\n37866\t47173\tSharps chapel\tTN\tUnion County\tH1\n37888\t47173\tWashburn\tTN\tUnion County\tH1\n37807\t47173\tMaynardville\tTN\tUnion County\tH1\n37825\t47173\tNew tazewell\tTN\tUnion County\tH1\n37779\t47173\tLuttrell\tTN\tUnion County\tH1\n37721\t47173\tCorryton\tTN\tUnion County\tH1\n37870\t47173\tSpeedwell\tTN\tUnion County\tH1\n37367\t47175\tPikeville\tTN\tVan Buren County\tH1\n38583\t47175\tSparta\tTN\tVan Buren County\tH1\n38585\t47175\tSpencer\tTN\tVan Buren County\tH1\n38559\t47175\tDoyle\tTN\tVan Buren County\tH1\n38581\t47175\tRock island\tTN\tVan Buren County\tH1\n37110\t47175\tMcminnville\tTN\tVan Buren County\tH1\n37166\t47177\tSmithville\tTN\tWarren County\tH1\n37357\t47177\tMorrison\tTN\tWarren County\tH1\n37394\t47177\tViola\tTN\tWarren County\tH1\n38550\t47177\tCampaign\tTN\tWarren County\tH1\n37190\t47177\tWoodbury\tTN\tWarren County\tH1\n38581\t47177\tRock island\tTN\tWarren County\tH1\n37110\t47177\tMcminnville\tTN\tWarren County\tH1\n37378\t47177\tSmartt\tTN\tWarren County\tH1\n37659\t47179\tJonesborough\tTN\tWashington County\tH1\n37605\t47179\tJohnson city\tTN\tWashington County\tH1\n37641\t47179\tChuckey\tTN\tWashington County\tH1\n37602\t47179\tJohnson city\tTN\tWashington County\tH1\n37615\t47179\tJohnson city\tTN\tWashington County\tH1\n37681\t47179\tLimestone\tTN\tWashington County\tH1\n37694\t47179\tWatauga\tTN\tWashington County\tH1\n37601\t47179\tJohnson city\tTN\tWashington County\tH1\n37690\t47179\tTelford\tTN\tWashington County\tH1\n37614\t47179\tJohnson city\tTN\tWashington County\tH1\n37604\t47179\tJohnson city\tTN\tWashington County\tH1\n37650\t47179\tErwin\tTN\tWashington County\tH1\n37663\t47179\tKingsport\tTN\tWashington County\tH1\n37656\t47179\tFall branch\tTN\tWashington County\tH1\n37686\t47179\tPiney flats\tTN\tWashington County\tH1\n37684\t47179\tMountain home\tTN\tWashington County\tH1\n38463\t47181\tIron city\tTN\tWayne County\tH1\n38425\t47181\tClifton\tTN\tWayne County\tH1\n38486\t47181\tWestpoint\tTN\tWayne County\tH1\n38475\t47181\tOlivehill\tTN\tWayne County\tH1\n38471\t47181\tLutts\tTN\tWayne County\tH1\n37096\t47181\tLinden\tTN\tWayne County\tH1\n38485\t47181\tWaynesboro\tTN\tWayne County\tH1\n38452\t47181\tCypress inn\tTN\tWayne County\tH1\n38450\t47181\tCollinwood\tTN\tWayne County\tH1\n38464\t47181\tLawrenceburg\tTN\tWayne County\tH1\n38226\t47183\tDukedom\tTN\tWeakley County\tH1\n38201\t47183\tMc kenzie\tTN\tWeakley County\tH1\n38242\t47183\tParis\tTN\tWeakley County\tH1\n38255\t47183\tSharon\tTN\tWeakley County\tH1\n38225\t47183\tDresden\tTN\tWeakley County\tH1\n38237\t47183\tMartin\t
